vi "NISE.local.Get Property Documentation.vi"(0 "SLSC Local in":refnum<class "SLSC Interface.lvclass">, 5 "property":refnum<k21>, 11 "error in (no error)":errorcluster) -> (4 "SLSC Local out":refnum<class "SLSC Interface.lvclass">, 6 "property out":refnum<k21>, 10 "Prop.Doc":string, 15 "error out":errorcluster)   [LabVIEW 2016, in "SLSC Interface.lvclass"]
uses:
  SLSC Interface Class/SLSC Interface.lvclass
  <resource>/objmgr/slsc.rc
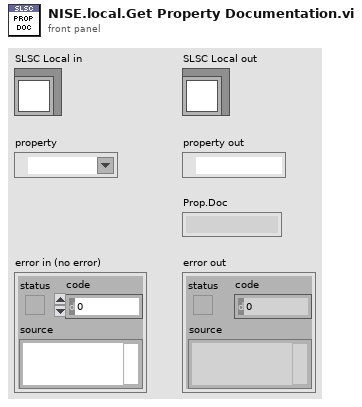
[diagram p1: front panel]
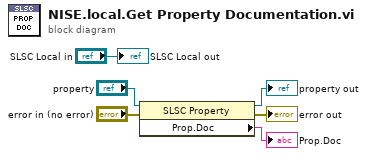
[diagram p0: block diagram]
diagram:
  n1 = property class="SLSC Property"(reference="property", error in="error in (no error)") -> (reference out=→"property out":refnum<k21>, error out=→"error out":errorcluster, "Prop.Doc"=→"Prop.Doc":string)
  "SLSC Local out" <- "SLSC Local in"
